vi "Apply View Matrix.vi"(10 "View Matrix":sgl[][](array[numeric]), 11 "Triangle in":T1) -> (3 "Triangle":T1)   [LabVIEW 2022 SP3, in "3D.lvlib"]
uses:
  3D.lvlib
  Triangle 3D.ctl
  Vector 3D.ctl
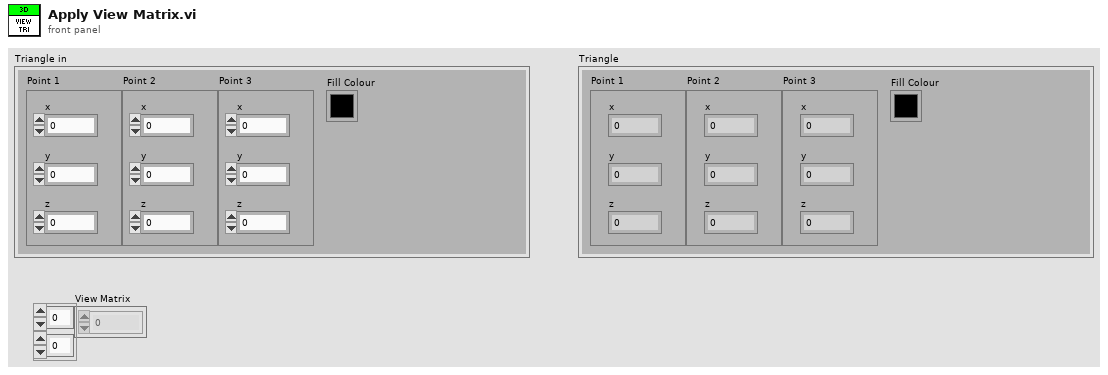
[diagram p1: front panel]
types:
  T1 = typedef "3D.lvlib/Triangle 3D.ctl" = cluster{"Point 1":T2, "Point 2":T2, "Point 3":T2, "Fill Colour":u32}
  T2 = typedef "3D.lvlib/Vector 3D.ctl" = cluster{"x":sgl, "y":sgl, "z":sgl}
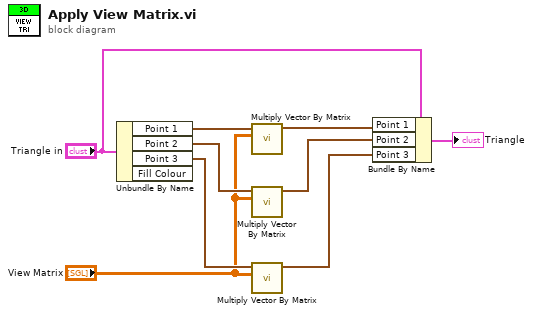
[diagram p0: block diagram]
diagram:
  n1 = Unbundle By Name("Triangle in") -> ("Point 1"=w7:T2, "Point 2"=w8:T2, "Point 3"=w9:T2)  [unwired: 1 out]
  n2 = call "Multiply Vector By Matrix.vi"("Matrix in"="View Matrix", "Vector 3D in"=w7) -> ("Vector 3D out"=w4:T2)  [unwired: 9 in]
  n3 = call "Multiply Vector By Matrix.vi"("Matrix in"="View Matrix", "Vector 3D in"=w8) -> ("Vector 3D out"=w2:T2)  [unwired: 9 in]
  n4 = call "Multiply Vector By Matrix.vi"("Matrix in"="View Matrix", "Vector 3D in"=w9) -> ("Vector 3D out"=w1:T2)  [unwired: 9 in]
  n5 = Bundle By Name(cluster="Triangle in", "Point 1"=w4, "Point 2"=w2, "Point 3"=w1) -> (→"Triangle":T1)
